vi "UE + DVR template.vi"() -> ()   [LabVIEW 2017]
uses:
  Error Handler/Controls/Error Event.ctl
  Error Handler/Controls/Error Type.ctl
  Controller/Controls/Controller Event.ctl
  Controller/Controls/Controller Command.ctl
  Controller/Controls/Controller Overhead.ctl
  Real-Time/RT Status.ctl
  Real-Time/RT Loop Status.ctl
  Controller/Controls/Controller DAQ Data.ctl
panel:
  in  "DAQ Data DVR":refnum<data-value>
  in  "Overhead DVR":refnum<data-value>
  in  "Command":refnum<user-event>
  in  "Stop DVR":refnum<data-value>
  in  "Stop":refnum<user-event>
  in  "Error":refnum<user-event>
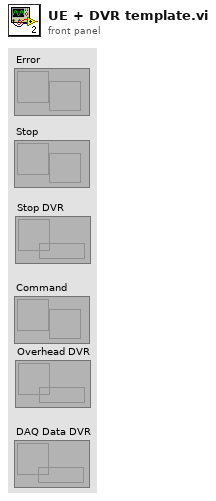
[diagram p1: front panel]
types:
  T1 = typedef "Controller DAQ Data.ctl" = cluster{"AOM data":dbl[], "AIMV data":dbl[], "AIMC data":dbl[], "DOM data":dbl[], "DIM data":dbl[], "AOM timestamp":dbl, "AIMV timestamp":dbl, "AIMC timestamp":dbl, "DOM timestamp":dbl, "DIM timestamp":dbl}
  T2 = typedef "Controller Overhead.ctl" = cluster{"Start":bool, "Numeric":dbl, "Blink CNTRLR1":bool, "Blink CNTRLR2":bool, "RT Status":T3}
  T3 = typedef "RT Status.ctl" = cluster{"Status TCL1":T4, "Status TCL2":T4, "Status NPL":T4, "Connected?":bool}
  T4 = typedef "RT Loop Status.ctl" = cluster{"Duration, us":dbl, "Late Counter":i32, "Timeout, us":u32}
  T5 = typedef "Controller Event.ctl" = cluster{"CMD":T6, "Data":variant}
  T6 = typedef "Controller Command.ctl" = enum16{"Idle", "Init", "Stop App", "Stop RT"}
  T7 = typedef "Error Event.ctl" = cluster{"ErrorType":T8, "error in":errorcluster}
  T8 = typedef "Error Type.ctl" = enum16{"Minor", "Critical"}
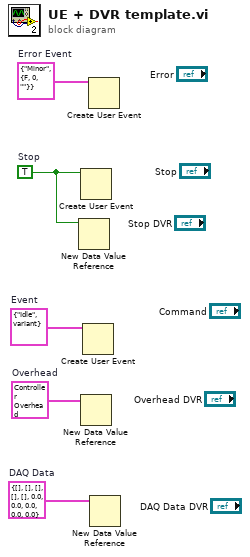
[diagram p0: block diagram]
diagram:
  w1 = T1 {"AOM data"=[], "AIMV data"=[], "AIMC data"=[], "DOM data"=[], "DIM data"=[], "AOM timestamp"=0.0, "AIMV timestamp"=0.0, "AIMC timestamp"=0.0, "DOM timestamp"=0.0, "DIM timestamp"=0.0}  # DAQ Data
  w2 = T2 {"Start"=FALSE, "Numeric"=0.0, "Blink CNTRLR1"=FALSE, "Blink CNTRLR2"=FALSE, "RT Status"={"Status TCL1"={"Duration, us"=0.0, "Late Counter"=0, "Timeout, us"=0}, "Status TCL2"={"Duration, us"=0.0, "Late Counter"=0, "Timeout, us"=0}, "Status NPL"={"Duration, us"=0.0, "Late Counter"=0, "Timeout, us"=0}, "Connected?"=FALSE}}  # Overhead
  w3 = T5 {"CMD"=enum."Idle", "Data"=variant}  # Event
  w4 = TRUE  # Stop
  w5 = T7 {"ErrorType"=enum."Minor", "error in"={"status"=FALSE, "code"=0, "source"=""}}  # Error Event
  n1 = New Data Value Reference(data value=w4) -> ()  [unwired: 1 in, 2 out]
  n2 = Create User Event(user event datatype=w4) -> ()  [unwired: 1 in, 2 out]
  n3 = New Data Value Reference(data value=w2) -> ()  [unwired: 1 in, 2 out]
  n4 = Create User Event(user event datatype=w3) -> ()  [unwired: 1 in, 2 out]
  n5 = Create User Event(user event datatype=w5) -> ()  [unwired: 1 in, 2 out]
  n6 = New Data Value Reference(data value=w1) -> ()  [unwired: 1 in, 2 out]
